vi "FM Modulation Demo (Single tone) - First(Phase-Locked Loop).vi"() -> ()   [LabVIEW 2013]
uses:
  <vilib>/addons/Modulation/Analog/MT Passband PLL.vi
  <vilib>/express/express analysis/Spectral/Block/exnSpectralBlock spectral measurements power poly.vi
  <vilib>/express/express analysis/Spectral/Block/exnSpectralBlock spectral measurements power DDT.vi
  <vilib>/express/express analysis/Spectral/XNode/ExpressSpectralMeasurementsBlockNode.xnode
  <vilib>/addons/Modulation/niAMT.lvlib
panel:
  in  "WAV SR":dbl=44100.0 caption="dt"
  in  "Mod. Freq.":dbl=2000.0 caption="Frequency"
  in  "LPF Cut-Off":dbl=10000.0 caption="Lower Cut-Off"
  in  "AWGN (dB)":dbl(slide)=0.6 caption="Standard deviation" scale=-20.0..30.0
  out "Comparision":dynamicdata(graph)
  out "Baseband":dynamicdata(graph)
  out "FM FFT":dynamicdata(graph)
  out "FM Wave":dynamicdata(graph)
  out "Estimated freq":dbl=1.0
  in  "Carrier Amp.":dbl=1.0 caption="Amplitude"
  in  "stop":bool
  in  "Frequency Deviation":dbl(slide)=1.0 scale=0.0..5.0
  in  "Carrier Freq.":dbl=100000.0 caption="Frequency"
  out "Recovered Signal":dynamicdata(graph)
  # "FM Modulation"
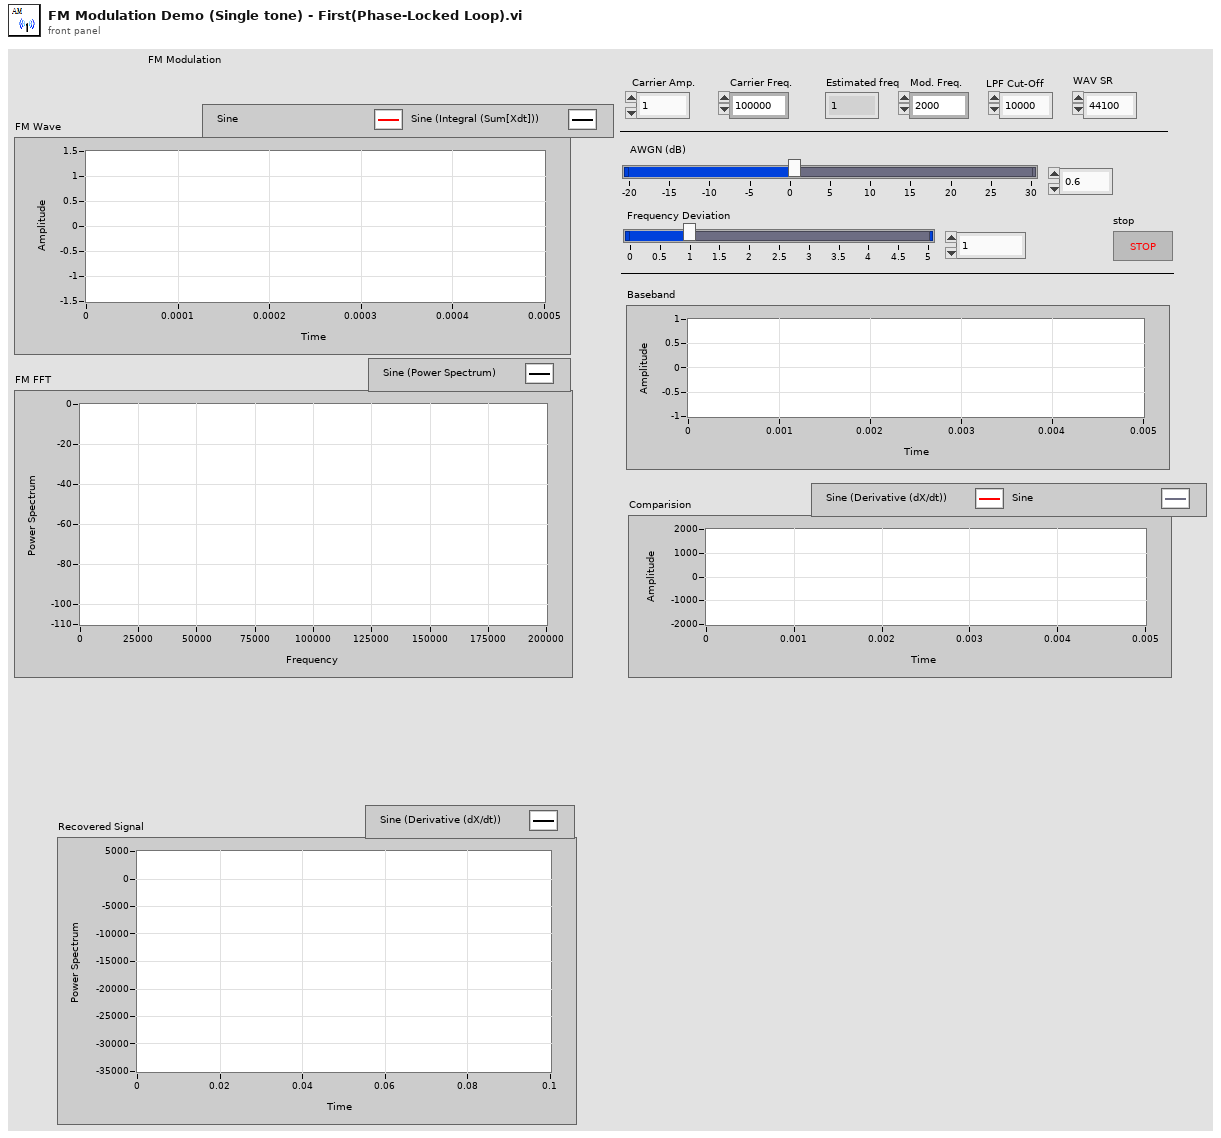
[diagram p1: front panel]
types:
  T1 = cluster{"averaging mode":u16, "weighting mode":u16, "number of averages":u32}
  T2 = cluster{"dB On (F)":bool, "unwrap phase (F)":bool, "convert to degree (F)":bool}
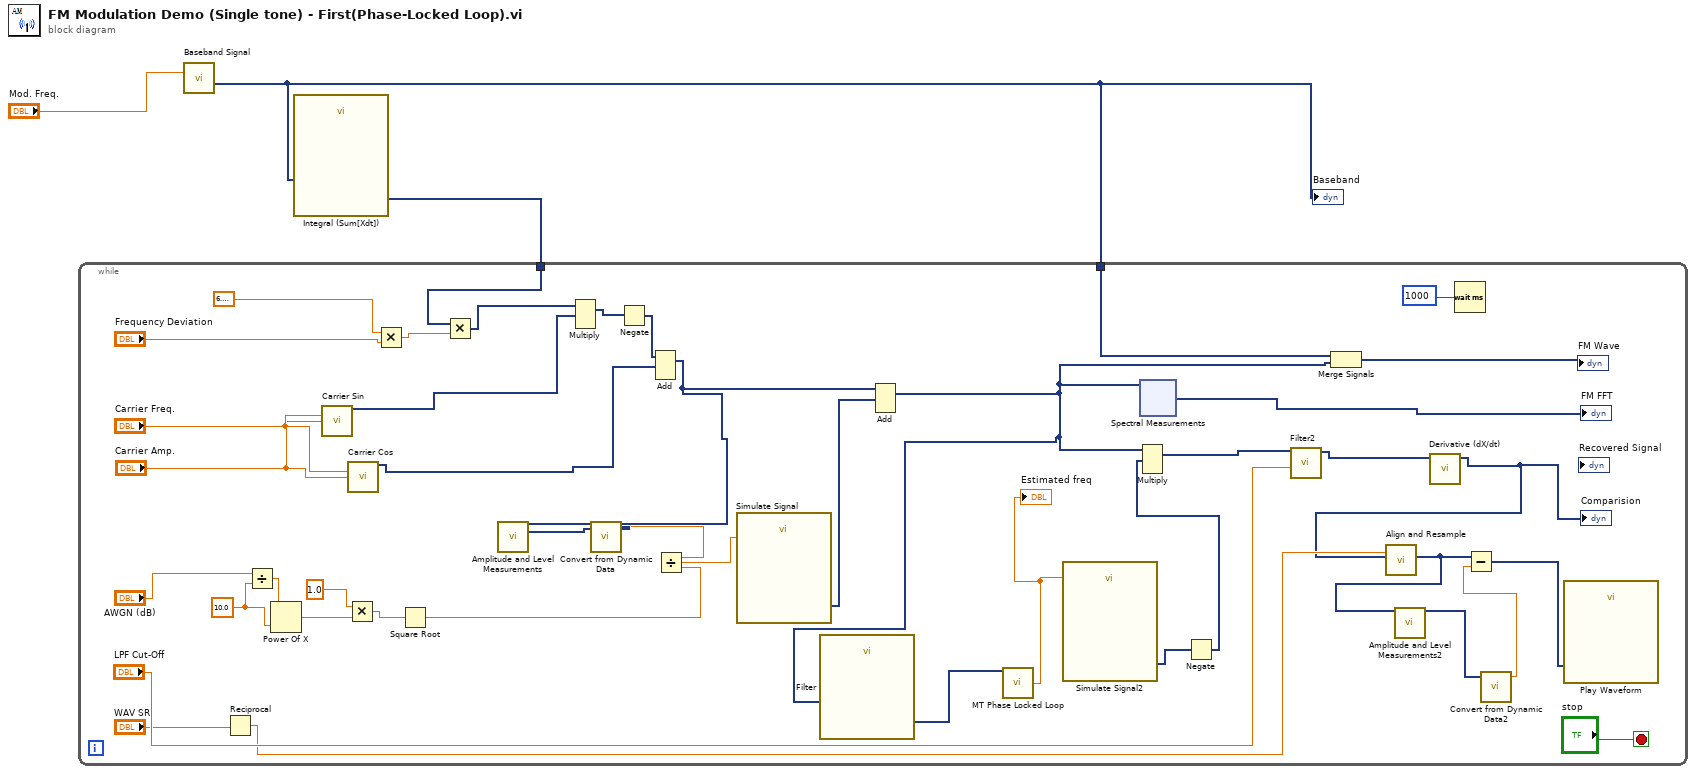
[diagram p0: block diagram]
diagram:
  n1 = call "Baseband Signal"("Frequency"="Mod. Freq.") -> ("Sine"=w2:dynamicdata)  [unwired: 13 in, 1 out]
  "Baseband" <- w2
  n2 = call "Integral (Sum[Xdt])"("Signals"=w2) -> ("Result"=w1:dynamicdata)  [unwired: 5 in, 1 out]
  n3 = while {
    tunnel: w2 -> [w24]
    tunnel: w1 -> [w28]
    stop <- "stop" stop-if-true
    w33 = 10.0
    n4 = Reciprocal(x="WAV SR") -> (1/x=w9:dbl)
    n5 = Divide(x="AWGN (dB)", y=w33) -> (x/y=w34:dbl)
    n6 = Power Of X(1:w33, 2:w34) -> (0:w32:dbl)
    n7 = call "Carrier Sin"("Frequency"="Carrier Freq.", "Amplitude"="Carrier Amp.") -> ("Sine"=w23:dynamicdata)  [unwired: 12 in, 1 out]
    n8 = Multiply(x=1.0, y=w32) -> (x*y=w40:dbl)
    n9 = call "Carrier Cos"("Frequency"="Carrier Freq.", "Amplitude"="Carrier Amp.") -> ("Sine"=w21:dynamicdata)  [unwired: 12 in, 1 out]
    n10 = Multiply(x=6.283185307179586, y="Frequency Deviation") -> (x*y=w29:dbl)
    n11 = Square Root(x=w40) -> (sqrt(x)=w38:dbl)
    n12 = Multiply(x=w28, y=w29) -> (x*y=w22:dynamicdata)
    n13 = Multiply(1:w23, 2:w22) -> (0:w20:dynamicdata)  [unwired: 1 in, 1 out]
    n14 = Negate(x=w20) -> (-x=w19:dynamicdata)
    n15 = Add(1:w21, 2:w19) -> (0:w25:dynamicdata)  [unwired: 1 in, 1 out]
    n16 = call "Amplitude and Level Measurements"("Signals"=w25) -> ("RMS"=w43:dynamicdata)  [unwired: 13 in, 1 out]
    n17 = call "Convert from Dynamic Data"("Dynamic Data Type"=w43) -> ("Scalar"=w39:dbl)  [unwired: 3 in]
    n18 = Divide(x=w39, y=w38) -> (x/y=w31:dbl)
    n19 = call "Simulate Signal"("Standard deviation"=w31) -> ("DC with Gaussian Noise"=w37:dynamicdata)  [unwired: 13 in, 1 out]
    n20 = Add(1:w37, 2:w25) -> (0:w18:dynamicdata)  [unwired: 1 in, 1 out]
    n21 = call "Filter"("Signal"=w18) -> ("Filtered Signal"=w17:dynamicdata)  [unwired: 9 in, 1 out]
    n22 = call-poly <vilib>:"MT Phase Locked Loop.vi"("passband waveform"=w17) -> ("estimated carrier frequency (Hz)"=w16:dbl)  [unwired: 10 in, 4 out]
    "Estimated freq" <- w16
    n23 = call "Simulate Signal2"("Frequency"=w16) -> ("Sine"=w15:dynamicdata)  [unwired: 13 in, 1 out]
    n24 = xnode "Spectral Measurements"("Signals"=w18) -> ("Power Spectrum"=→"FM FFT":dynamicdata)  [unwired: 1 in, 1 out]
    n25 = Negate(x=w15) -> (-x=w14:dynamicdata)
    n26 = Multiply(1:w14, 2:w18) -> (0:w13:dynamicdata)  [unwired: 1 in, 1 out]
    n27 = call "Filter2"("Lower Cut-Off"="LPF Cut-Off", "Signal"=w13) -> ("Filtered Signal"=w11:dynamicdata)  [unwired: 8 in, 1 out]
    n28 = Merge Signals(w24, w18) -> (→"FM Wave":dynamicdata)
    n29 = call "Derivative (dX/dt)"("Signals"=w11) -> ("Result"=w4:dynamicdata)  [unwired: 5 in, 1 out]
    "Comparision" <- w4
    n30 = call "Align and Resample"("dt"=w9, "Signals"=w4) -> ("Resampled Signals"=w8:dynamicdata)  [unwired: 7 in, 2 out]
    n31 = call "Amplitude and Level Measurements2"("Signals"=w8) -> ("Mean (DC)"=w7:dynamicdata)  [unwired: 13 in, 1 out]
    n32 = Wait (ms)(milliseconds to wait=1000) -> ()  [unwired: 1 out]
    n33 = call "Convert from Dynamic Data2"("Dynamic Data Type"=w7) -> ("Scalar"=w6:dbl)  [unwired: 3 in]
    n34 = Subtract(x=w8, y=w6) -> (x-y=w5:dynamicdata)
    n35 = call "Play Waveform"("Data"=w5) -> ()  [unwired: 18 in, 1 out]
  }
